vi "Execute.vi"(8 "error in (no error)":errorcluster, 9 "System in":refnum<class "System.lvclass">, 10 "Command in":refnum<class "Command.lvclass">, 11 "GrabberArms-ExtendingState in":refnum<class "GrabberArms-ExtendingState.lvclass">) -> (0 "error out":errorcluster, 2 "Next State":refnum<class "State.lvclass">, 3 "GrabberArms-ExtendingState out":refnum<class "GrabberArms-ExtendingState.lvclass">)   [LabVIEW 2013, in "GrabberArms-ExtendingState.lvclass"]
uses:
  GrabberArms-ExtendingState.lvclass
  Commands/Command/Command.lvclass
  Systems/System/System.lvclass
  State/State.lvclass
  Systems/GrabberArms/GrabberArms.lvclass
  GA-Extended-State/GrabberArms-ExtendedState.lvclass
  Robot Global Data.vi
panel:
  in  "Test Button":bool
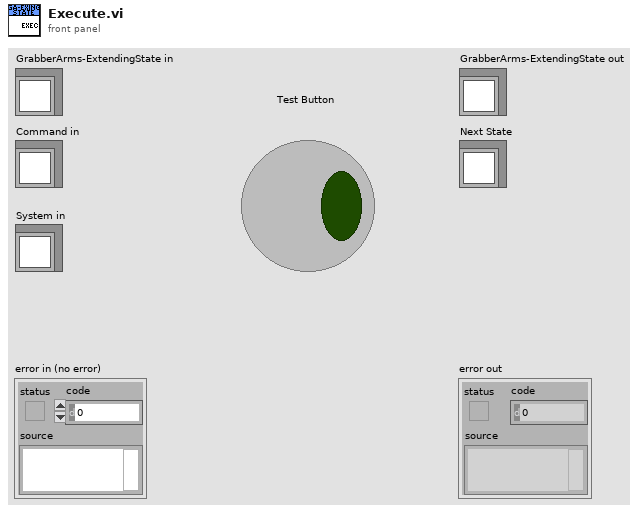
[diagram p1: front panel]
types:
  T1 = typedef "WPI_DigitalInputDevRef.ctl" = cluster{"DevStatus":errorcluster, "DIO Channel":T2, "Digital Module":T3}
  T2 = typedef "FPGA_DIOChannel.ctl" = enum8{"DIO 1", "DIO 2", "DIO 3", "DIO 4", "DIO 5", "DIO 6", "DIO 7", "DIO 8", "DIO 9", "DIO 10", "DIO 11", "DIO 12", "DIO 13", "DIO 14", "Invalid"}
  T3 = typedef "FPGA_TypedefDigitalModule.ctl" = enum16{"Digital Module 1", "Digital Module 2"}
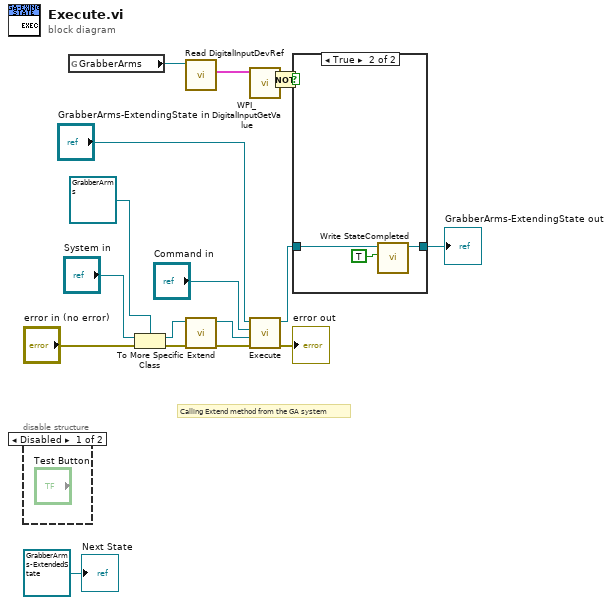
[diagram p0: block diagram]
diagram:
  # "Calling Extend method from the GA system"
  n1 = disable-structure shown="Disabled" {
    frame Disabled {
    }
    frame Enabled {
    }
  }
  n2 = global read "Robot Global Data.vi" "GrabberArms"() -> (w3:refnum<class "GrabberArms.lvclass">)
  n3 = To More Specific Class(target class=refnum<class "GrabberArms.lvclass"> refnum ("GrabberArms.lvclass"), reference="System in", error in="error in (no error)") -> (specific class reference=w12:refnum<class "GrabberArms.lvclass">, error out=w9:errorcluster)
  n4 = call-dynamic "Read DigitalInputDevRef.vi"("GrabberArms in"=w3) -> ("DigitalInputDevRef"=w2:T1)  [unwired: 8 in, 2 out]
  n5 = call-dynamic "Extend.vi"("error in (no error)"=w9, "GrabberArms in"=w12) -> ("error out"=w8:errorcluster, "GrabberArms out"=w11:refnum<class "GrabberArms.lvclass">)  [unwired: 8 in]
  n6 = call <vilib>:"WPI_DigitalInputGetValue.vi"("DigitalInputDevRef"=w2) -> ("Value"=w4:bool)  [unwired: 8 in, 2 out]
  n7 = call-parent "Execute.vi"("error in (no error)"=w8, "System in"=w11, "Command in"="Command in", "State in"="GrabberArms-ExtendingState in") -> ("error out"=→"error out":errorcluster, "State out"=w5:refnum<class "GrabberArms-ExtendingState.lvclass">)  [unwired: 5 in, 1 out]
  n8 = Not(x=w4) -> (.not. x?=w1:bool)
  n9 = case shown="True" w1 {
    tunnel: w5 -> [w18 w21]
    tunnel: [w18 w20] -> w6
    frame False {
    }
    frame True {
      n10 = call-dynamic "Write StateCompleted.vi"("StateCompleted"=TRUE, "State in"=w21) -> ("State out"=w20:refnum<class "GrabberArms-ExtendingState.lvclass">)  [unwired: 8 in, 1 out]
    }
  }
  "GrabberArms-ExtendingState out" <- w6
  "Next State" <- refnum<class "GrabberArms-ExtendedState.lvclass"> refnum ("GrabberArms-ExtendedState.lvclass")
